vi "Motor Schedule Reader.vi"() -> ()   [LabVIEW 2020]
uses:
  <vilib>/platform/TimedLoop/XDataNode/XDataNode.xnode
  <vilib>/Platform/TimedLoop/XDataNode/nitl_modes.ctl
  <vilib>/Platform/TimedLoop/XDataNode/XDNodeRunTimeDep.lvlib
  <vilib>/Platform/TimedLoop/XDataNode/wakeup.ctl
  <vilib>/Platform/TimedLoop/XDataNode/timing_clust.ctl
  <vilib>/Analysis/NI_AALBase.lvlib
  <vilib>/Utility/file.llb/Read Delimited Spreadsheet (string).vi
panel:
  out "Numeric 2":i32
  out "subarray":string[][](array[string])
  out "all rows":string[][](array[string])
  in  "file path (dialog if empty)":path
  out "output cluster":cluster{dbl[], dbl[]}
  out "XY Graph":cluster{"sine wave":dbl[], "sine wave":dbl[]}[](graph)
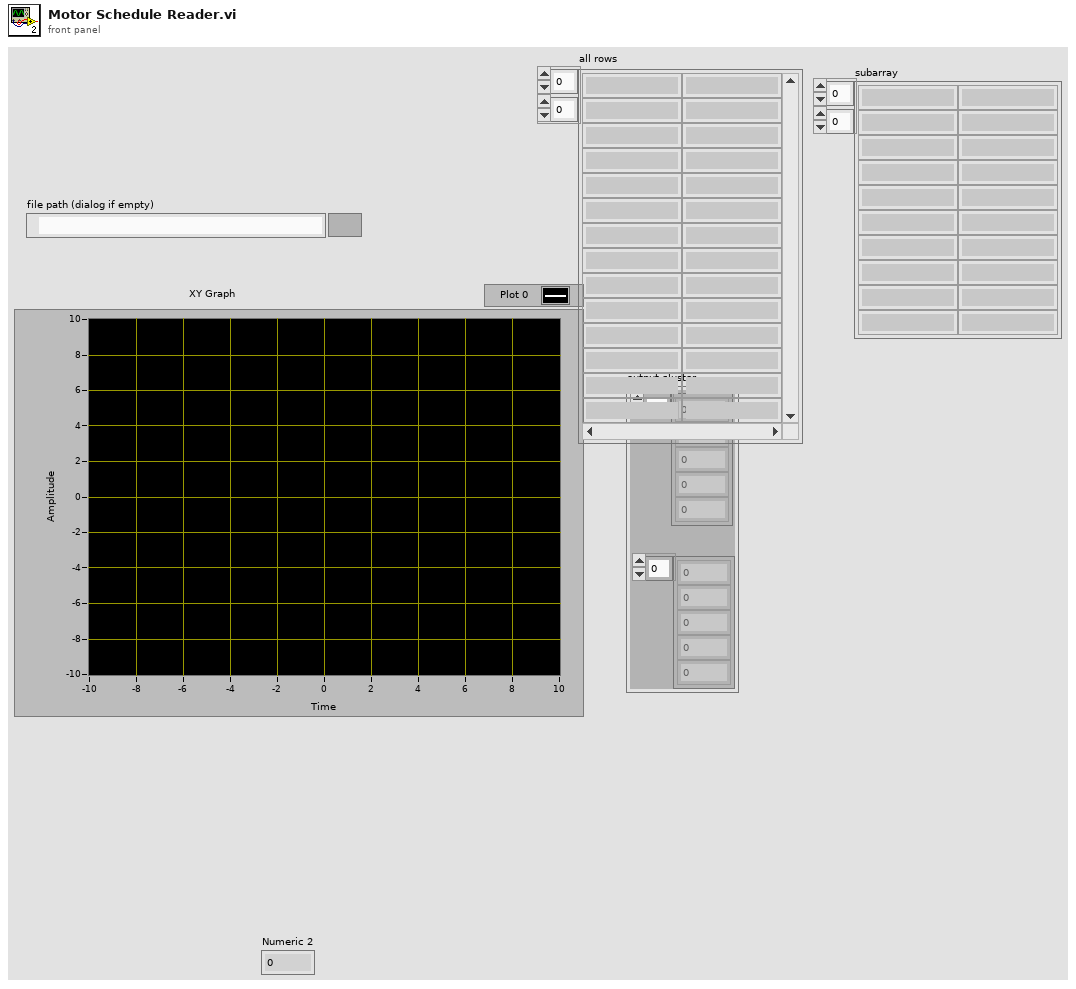
[diagram p1: front panel]
types:
  T1 = typedef "XDNodeRunTimeDep.lvlib/timing_clust.ctl" = cluster{"Expected End [f-1]":u64, "Actual End [f-1]":u64, "Finished Late? [f-1]":bool, "Expected End [i-1]":u64, "Actual End [i-1]":u64, "Finished Late? [i-1]":bool, "Expected Start [i]":u64, "Actual Start [i]":u64, "Expected Start [f]":u64, "Actual Start [f]":u64, "Source Name":string, "Structure Name":string, "Period":i64, "Deadline":i64, "Offset":i64, "Start":i64, "Priority":i32, "Timeout":i32, "Mode":T2, "Wakeup Reason":T3, "Error":errorcluster, "Source Type":string, "Secondary Source Type":string, "Global End Time":u64, "Global Start Time":u64, "Frame Duration":u64, "Iteration Duration":u64, "Assigned CPU":i32, "I/O Scan Engine Mode":u32}
  T2 = typedef "XDNodeRunTimeDep.lvlib/nitl_modes.ctl" = enum32{"No Change", "Process missed periods, maintain original phase", "Discard missed periods, maintain original phase", "Process missed periods, ignore original phase", "Discard missed periods, ignore original phase"}
  T3 = typedef "XDNodeRunTimeDep.lvlib/wakeup.ctl" = enum32{"Normal", "Aborted", "Asynchronous wakeup", "Timing source error", "Timed loop error", "Timeout"}
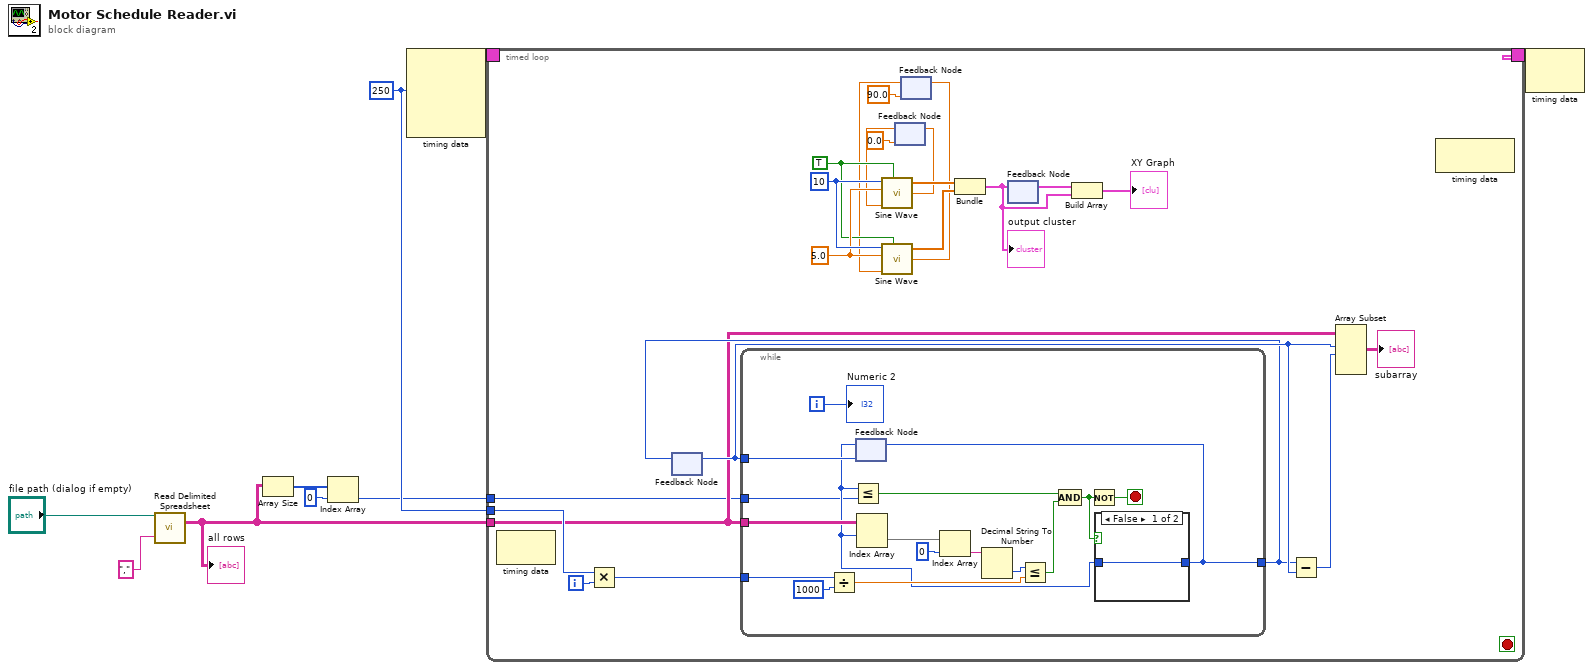
[diagram p0: block diagram]
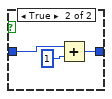
[diagram p2: hidden frame]
diagram:
  w7 = i64 250 ("Period")
  n1 = call-poly <vilib>:"Read Delimited Spreadsheet.vi"("file path (dialog if empty)"="file path (dialog if empty)", "delimiter (\\t)"="," ("delimiter (\\t)")) -> ("all rows"=w2:string[][])  [unwired: 8 in, 5 out]
  "all rows" <- w2
  n2 = Array Size(array=w2) -> (size(s)=w4:i32[])
  n3 = Index Array(array=w4, index=0) -> (element=w1:i32)
  n4 = node-c288(w7) -> (w9:T1)  [unwired: 3 in]
  n5 = timed-loop {
    timing: w9 -> [_]
    timing-out: [_] -> w8
    tunnel: w7 -> [w18]
    tunnel: w2 -> [w11]
    tunnel: w1 -> [w10]
    i -> [w17]
    stop <- _ stop-if-true
    w28 = TRUE ("reset phase")
    w30 = 5.0 ("amplitude")
    w31 = 10 ("samples")
    n6 = node-c288() -> ()  [unwired: 1 in, 1 out]
    n7 = Multiply(x=w18, y=w17) -> (x*y=w13:i64)
    n8 = feedback #1() -> (w14:i32)  [unwired: 1 in]
    n9 = while {
      tunnel: [w38] -> w12
      tunnel: w11 -> [w49]
      tunnel: w13 -> [w46]
      tunnel: w14 -> [w40]
      tunnel: w10 -> [w33]
      i -> [w39]
      stop <- w41 stop-if-true
      n10 = Divide(x=w46, y=i64 1000 ("x")) -> (x/y=w42:dbl)
      n11 = feedback #2(w40) -> (w35:i32)
      n12 = Less Or Equal?(x=w35, y=w33) -> (x <= y?=w34:bool)
      n13 = Index Array(array=w49, index (row)=w35) -> (element=w48:string[])  [unwired: 1 in]
      n14 = Index Array(array=w48, index=0) -> (element=w44:string)
      n15 = Decimal String To Number(string=w44) -> (number=w43:i32)  [unwired: 2 in, 1 out]
      n16 = Less Or Equal?(x=w43, y=w42) -> (x <= y?=w36:bool)
      n17 = Compound Arithmetic op=AND(w34, w36) -> (w37:bool)
      n18 = Not(x=w37) -> (.not. x?=w41:bool)
      n19 = case shown="False" w37 {
        tunnel: [w50 w52] -> w38
        tunnel: w35 -> [w50 w51]
        frame False {
        }
        frame True {
          n20 = Add(x=w51, y=1) -> (x+y=w52:i32)
        }
      }
      n21 = feedback-in #2(w38) -> ()
      "Numeric 2" <- w39
    }
    n22 = feedback-in #1(w12) -> ()
    n23 = feedback #3(0.0 ("phase out")) -> (w22:dbl)
    n24 = call <vilib>:"Sine Wave.vi"("samples"=w31, "amplitude"=w30, "phase in"=w22, "reset phase"=w28) -> ("sine wave"=w32:dbl[], "phase out"=w23:dbl)  [unwired: 1 in, 1 out]
    n25 = feedback-in #3(w23) -> ()
    n26 = feedback #4(90.0 ("phase out")) -> (w25:dbl)
    n27 = call <vilib>:"Sine Wave.vi"("samples"=w31, "amplitude"=w30, "phase in"=w25, "reset phase"=w28) -> ("sine wave"=w29:dbl[], "phase out"=w26:dbl)  [unwired: 1 in, 1 out]
    n28 = feedback-in #4(w26) -> ()
    n29 = Bundle("sine wave"=w32, "sine wave"=w29) -> (w20:cluster{"sine wave":dbl[], "sine wave":dbl[]})  [unwired: 1 in]
    "output cluster" <- w20
    n30 = feedback-in #5(w20) -> ()
    n31 = feedback #5() -> (w21:cluster{"sine wave":dbl[], "sine wave":dbl[]})  [unwired: 1 in]
    n32 = Build Array(w21, w20) -> (→"XY Graph":cluster{"sine wave":dbl[], "sine wave":dbl[]}[])
    n33 = Subtract(x=w12, y=w14) -> (x-y=w16:i32)
    n34 = Array Subset(array=w11, index (row)=w14, length (row)=w16) -> (→"subarray":string[][])  [unwired: 2 in]
    n35 = node-c288() -> ()  [unwired: 1 in, 1 out]
  }
  n36 = node-c288(w8) -> ()  [unwired: 1 out]
